vi "test2DArray.vi"(8 "error in (no error)":errorcluster) -> (0 "error out":errorcluster)   [LabVIEW 2019, in "AssertionTest.lvlib" / "AssertCount.lvlib"]
uses:
  AssertCount.lvlib
  Assertion/Assertion.lvlib
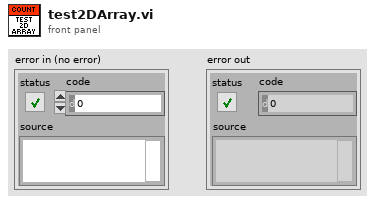
[diagram p1: front panel]
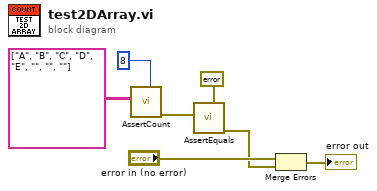
[diagram p0: block diagram]
diagram:
  n1 = call "AssertCount.vi"("Expected"=8, "Haystack"=string[][] [["A", "B", "C", "D"], ["E", "", "", ""]]) -> ("error out"=w1:errorcluster)  [unwired: 9 in]
  n2 = call "AssertEquals.vi"("Expected"=errorcluster {"status"=FALSE, "code"=0, "source"=""} ("error constant"), "Actual"=w1) -> ("error out"=w2:errorcluster)  [unwired: 9 in]
  n3 = Merge Errors("error in (no error)", w2) -> (→"error out":errorcluster)
